vi "Exp11 Controle Proporcional Derivativo_exercício.vi"() -> ()   [LabVIEW 2017]
doc: "This example demonstrates a simple PID position controller for a Quanser SRV-02 plant."
uses:
  <vilib>/Simulation/Scripting/Companion Diagram/SimConfigNode/SimParams.ctl
  <vilib>/Simulation/Scripting/Companion Diagram/SimConfigNode/_simSolvers.ctl
  <vilib>/Simulation/Implementation/Shared/SIMSCR Execution Mode.ctl
  <vilib>/Platform/TimedLoop/XDataNode/timing_clust.ctl
  <vilib>/Platform/TimedLoop/XDataNode/nitl_modes.ctl
  <vilib>/Platform/TimedLoop/XDataNode/wakeup.ctl
  <vilib>/Simulation/Param Hierarchy/Typedefs/SIMPH Param Control Actions.ctl
  <vilib>/Simulation/Implementation/Shared/NILVSim_ParamChanged.vi
  <vilib>/Simulation/Implementation/Shared/NILVSim_FinishedLate.vi
  <vilib>/Simulation/Implementation/Shared/NILVSIM_BeginStep.vi
  <vilib>/Simulation/SignalArithmetic/Implementation/NILVSim Gain.llb/SIM Gain (scalar).vi
  <vilib>/Simulation/Utility/Implementation/NILVSim Collector.llb/SIM Collector (scalar).vi
  <vilib>/Simulation/ContinuousLinear/Implementation/NILVSim Derivative.llb/SIM derivative (scalar).vi
  <vilib>/Simulation/DataSources/Implementation/NILVSim Pulse Generator.llb/SIM Pulse Generator (scalar).vi
  <vilib>/Simulation/Nonlinear/Implementation/NILVSim Saturation.llb/SIM Saturation (scalar).vi
  <vilib>/Simulation/Utility/Implementation/SIM Halt.vi
  <vilib>/Simulation/ContinuousLinear/Implementation/NILVSim Transfer Function.llb/SIM Transfer Function Distributor (SISO).vi
  <vilib>/Simulation/ContinuousLinear/Implementation/NILVSim Transfer Function.llb/SIM Transfer Function Collector (SISO).vi
  <vilib>/Simulation/Implementation/Shared/NILVSim_Manager.vi
  <vilib>/Utility/error.llb/Clear Errors.vi
  <vilib>/Simulation/Implementation/Shared/NILVSim_FinalizeModel.vi
  <vilib>/Simulation/Utility/Implementation/NILVSim Collector.llb/NILVSim Collector core (scalar).vi
  <vilib>/Simulation/Implementation/Shared/SIM Unbundle Sim Info.vi
  <vilib>/Simulation/Implementation/Shared/SIMSH Read Queue.vi
  <vilib>/Simulation/Implementation/Shared/NILVSim_Initialize.vi
  <vilib>/Simulation/Utility/Implementation/NILVSim Get Time and IsAcceptedStep.vi
  <vilib>/Simulation/Implementation/Shared/NILVSim_GetModelError.vi
  <vilib>/Simulation/Implementation/Shared/SIM Bundle Sim Info.vi
  <vilib>/addons/System Identification/Parametric Estimation.llb/SI Estimate Continuous Transfer Function Model (SISO Array).vi
  <vilib>/addons/Control Design/_Model Construction/Model Creation.llb/Model Creation SubVI/cd_Create Transfer Function Model.vi
  <vilib>/addons/Control Design/_Utility/Model Viewer.llb/Model Viewer SubVI/cd_Draw Transfer Function Equation (TF).vi
  <vilib>/Simulation/Scripting/Companion Diagram/SimConfigNode/SimDog.xnode
  <vilib>/Quanser/Rapid Control Prototyping Toolkit/hardware/HIL Immediate IO/_TypeSpecific/CL HIL Read Encoder (Scalar).vi
  <vilib>/Quanser/Rapid Control Prototyping Toolkit/hardware/HIL Immediate IO/CL HIL Read.vi
  <vilib>/Quanser/Rapid Control Prototyping Toolkit/hardware/HIL Immediate IO/_TypeSpecific/CL HIL Write Analog (Scalar).vi
  <vilib>/Quanser/Rapid Control Prototyping Toolkit/hardware/HIL Immediate IO/CL HIL Write.vi
  <vilib>/Platform/TimedLoop/XDataNode/XDataNode.xnode
  <vilib>/Simulation/Implementation/XNodeFramework/SimXNode/SimX.xnode
  <vilib>/addons/System Identification/NI_SysID.lvlib
  <vilib>/addons/Control Design/_Utility/NI_CD_Model Viewer.lvlib
  <vilib>/addons/Control Design/_Model Construction/NI_LinSys_Model Creation.lvlib
  <vilib>/Simulation/ContinuousLinear/Implementation/NILVSim Transfer Function.llb/SIM Transfer Function (SISO).vi
  <vilib>/Platform/TimedLoop/XDataNode/XDNodeRunTimeDep.lvlib
  <vilib>/Simulation/Implementation/Shared/NI_SIM_Implementation.lvlib
panel:
  in  "orders of transfer function model":cluster{" num order":i32, "den order":i32}={" num order"=1, "den order"=2}
  out "Equation":picture
  in  "Stop Button":bool
  in  "Kd":dbl(knob)=0.15 scale=0.0..1.0
  in  "Kp":dbl(knob)=2.5 scale=1.0..4.0
  out "XY Graph":cluster{"Time":dbl[], "Signal":dbl[]}[](graph)
  out "Posição [rad]":T1(graph)={"output"=3.1415, "output"=3.1569324614686494, "Result"=3.1415268333537414}
  out "encoder counts":i32=1029
  out "Error":errorcluster
  # "Controle PD"
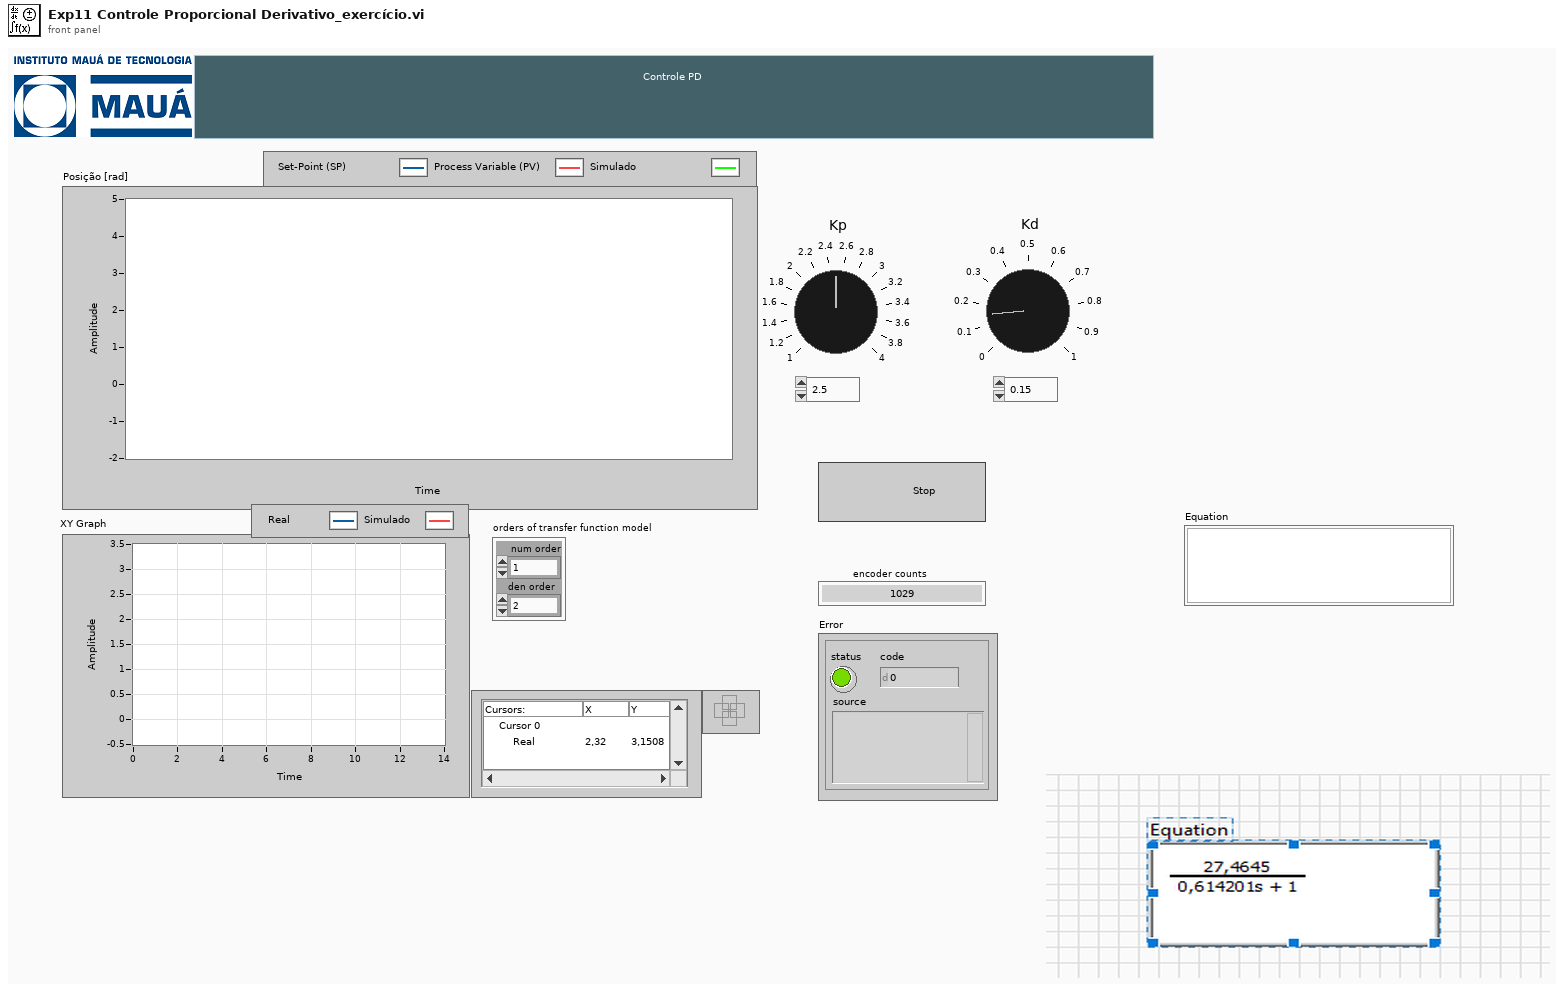
[diagram p1: front panel]
types:
  T1 = cluster{"output":dbl, "output":dbl, "Result":dbl}
  T2 = typedef "NI_LinSys_Model Typedefs.lvlib/CD Transfer Function Model (MIMO).ctl" = cluster{"properties":T3, "transfer function(s)":T4[][]}
  T3 = typedef "NI_LinSys_Model Typedefs.lvlib/CD General Elements.ctl" = cluster{"Model name":string, "Input names":string[], "Output names":string[], "Input Delays":dbl[], "Output Delays":dbl[], "Sampling Time":dbl, "Notes":string}
  T4 = typedef "NI_LinSys_Model Typedefs.lvlib/CD Transfer Function Model (SISO).ctl" = cluster{"Numerator":dbl[], "Denominator":dbl[], "delay":dbl}
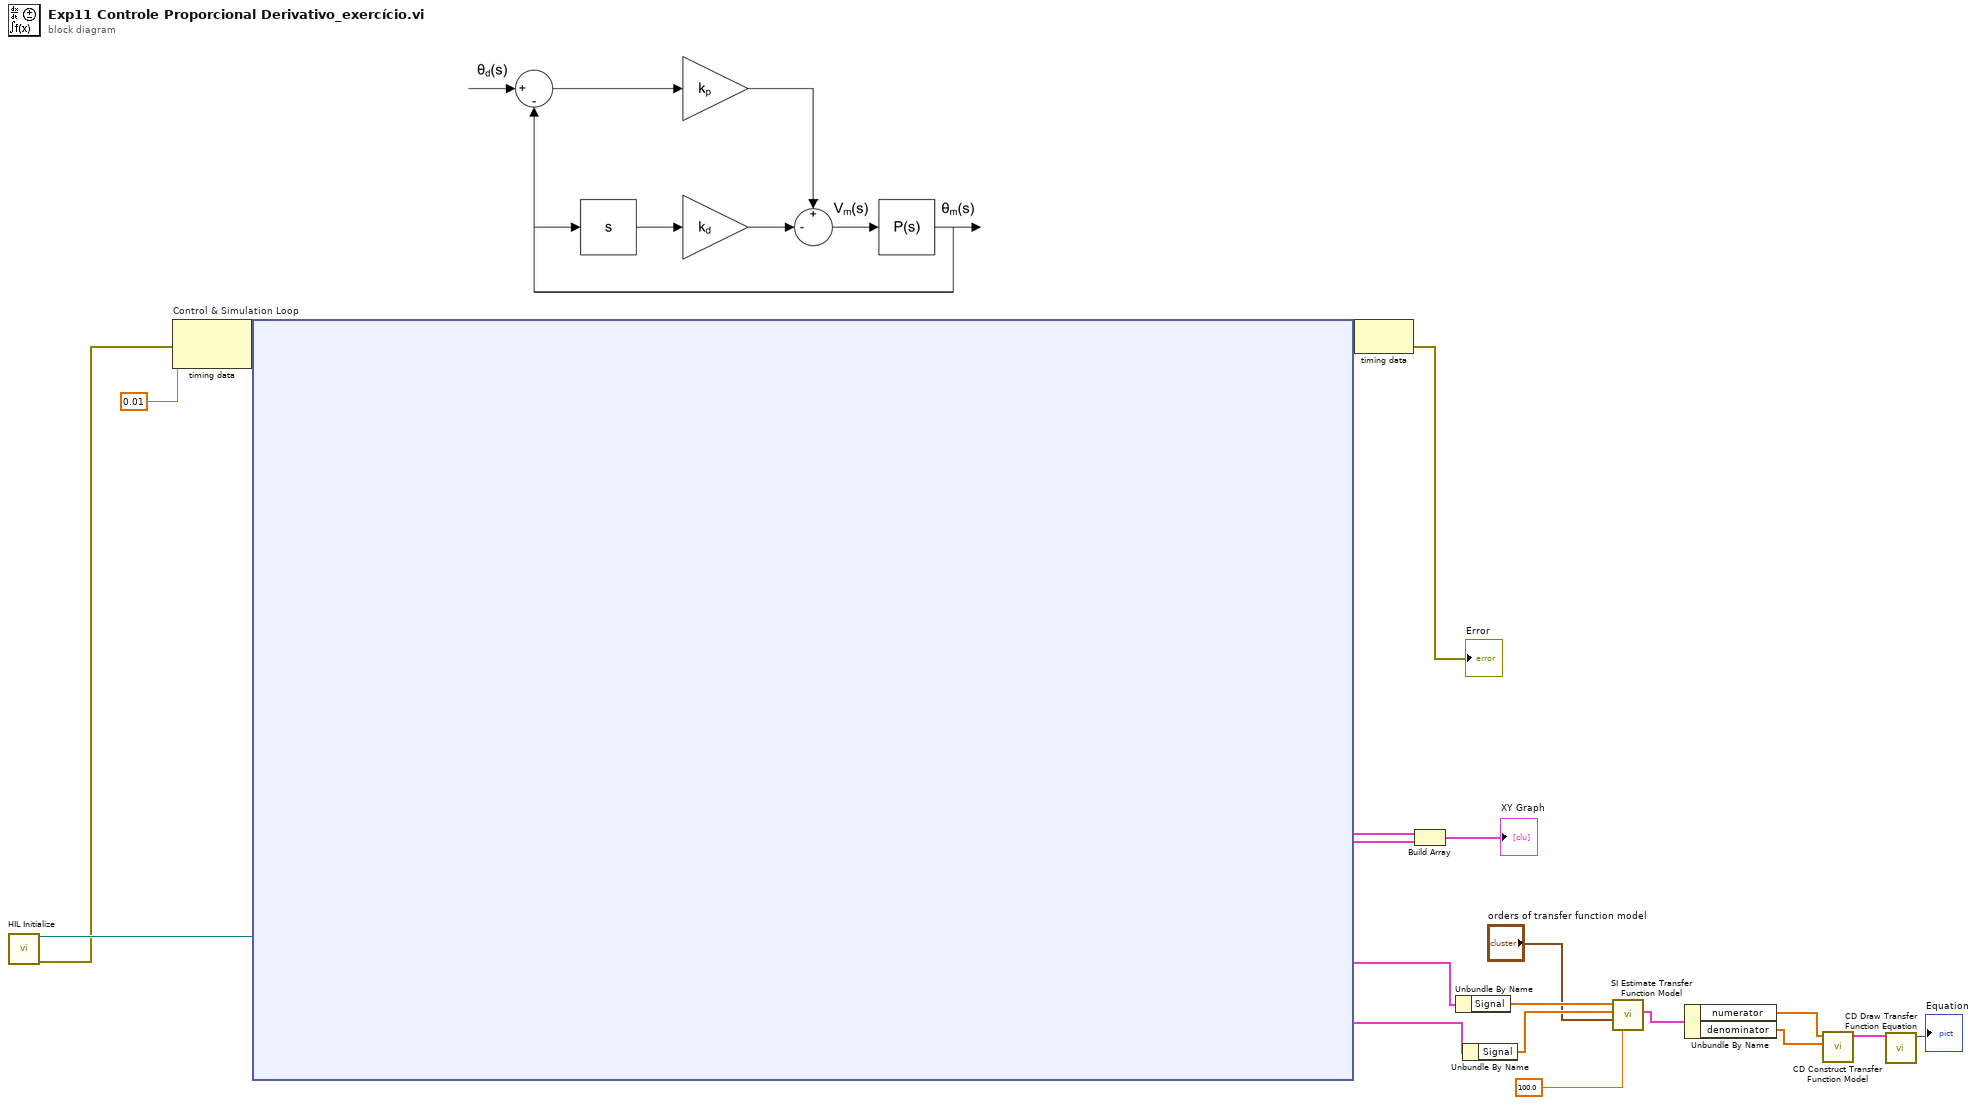
[diagram p0: block diagram]
diagram:
  n1 = call "HIL Initialize"() -> ("board out"=w18:refnum<class "HIL Board.lvclass">, "error out"=w15:errorcluster)  [unwired: 14 in]
  n2 = node-c288(w15, 0.01 ("Step Size (s)")) -> (w20:variant)
  n3 = node-c254 "Control & Simulation Loop"(w20, w18) -> (w19:variant, w14:cluster{"Time":dbl[], "Signal":dbl[]}, w12:cluster{"Time":dbl[], "Signal":dbl[]}, w2:cluster{"Time":dbl[], "Signal":dbl[]}, w1:cluster{"Time":dbl[], "Signal":dbl[]})
  n4 = node-c288(w19) -> (→"Error":errorcluster)
  n5 = Build Array "Build Array"(w14, w12) -> (→"XY Graph":cluster{"Time":dbl[], "Signal":dbl[]}[])
  n6 = Unbundle By Name(w2) -> ("Signal"=w5:dbl[])
  n7 = Unbundle By Name(w1) -> ("Signal"=w4:dbl[])
  n8 = call-poly <vilib>:"SI Estimate Transfer Function Model.vi"("sampling rate (Hz)"=100.0, "orders of transfer function model"="orders of transfer function model", "response signal"=w4, "stimulus signal"=w5) -> ("coefficients of transfer function model"=w11:cluster{"numerator":dbl[], "denominator":dbl[]})  [unwired: 4 in, 3 out]
  n9 = Unbundle By Name(w11) -> ("numerator"=w10:dbl[], "denominator"=w9:dbl[])
  n10 = call-poly <vilib>:"CD Construct Transfer Function Model.vi"("Denominator"=w9, "Numerator"=w10) -> ("Transfer Function Model"=w8:T2)  [unwired: 8 in, 1 out]
  n11 = call-poly <vilib>:"CD Draw Transfer Function Equation.vi"("Transfer Function Model"=w8) -> ("Equation"=→"Equation":picture)  [unwired: 8 in, 2 out]
